vi "Photoeye.vi"(11 "Update":bool) -> (3 "BeamBroken?":bool)   [LabVIEW 2015]
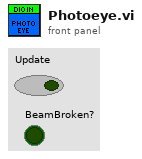
[diagram p1: front panel]
types:
  T1 = typedef "WPI_DigitalInputDevRef.ctl" = cluster{"DevStatus":errorcluster, "DIO Channel":T2}
  T2 = typedef "FPGA_DIOChannel.ctl" = enum8{"DIO 0", "DIO 1", "DIO 2", "DIO 3", "DIO 4", "DIO 5", "DIO 6", "DIO 7", "DIO 8", "DIO 9", "DIO MXP 0", "DIO MXP 1", "DIO MXP 2", "DIO MXP 3", "DIO MXP 4", "DIO MXP 5", "DIO MXP 6", "DIO MXP 7", "DIO MXP 8", "DIO MXP 9", "DIO MXP 10", "DIO MXP 11", "DIO MXP 12", "DIO MXP 13", "DIO MXP 14", "DIO MXP 15", "Invalid"}
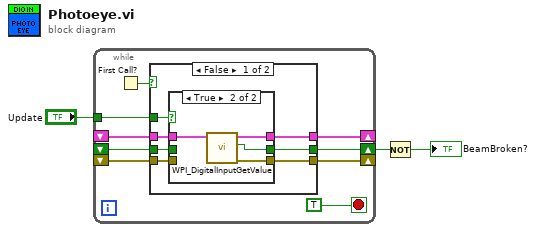
[diagram p0: block diagram]
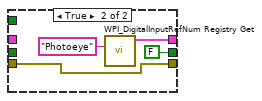
[diagram p3: hidden frame]
diagram:
  n1 = while {
    tunnel: "Update" -> [w10]
    shift-right: [w9] -> _
    shift-left: _ -> [w8]
    shift-right: [w7] -> w2
    shift-left: _ -> [w6]
    shift-right: [w5] -> _
    shift-left: _ -> [w4]
    stop <- TRUE stop-if-true
    n2 = First Call?() -> (First Call?: T/F=w11:bool)
    n3 = case shown="False" w11 {
      tunnel: w10 -> [w19 _]
      tunnel: [w18 w28] -> w9
      tunnel: w8 -> [w17 _]
      tunnel: [w16 FALSE ("Value")] -> w7
      tunnel: w6 -> [w15 _]
      tunnel: [w14 w27] -> w5
      tunnel: w4 -> [w13 w27]
      frame False {
        n4 = case shown="True" w19 {
          tunnel: [w22 w25] -> w18
          tunnel: w17 -> [w22 w26]
          tunnel: [w21 w23] -> w16
          tunnel: w15 -> [w21 _]
          tunnel: [w20 w24] -> w14
          tunnel: w13 -> [w20 _]
          frame False {
          }
          frame True {
            n5 = call <vilib>:"WPI_DigitalInputGetValue.vi"("DigitalInputDevRef"=w26) -> ("error out"=w24:errorcluster, "Value"=w23:bool, "DigitalInputDevRef"=w25:T1)  [unwired: 8 in]
          }
        }
      }
      frame True {
        n6 = call <vilib>:"WPI_DigitalInputRefNum Registry Get.vi"("refnum name"="Photoeye") -> ("DigitalInputDevRef"=w28:T1)  [unwired: 9 in, 1 out]
      }
    }
  }
  n7 = Not(x=w2) -> (.not. x?=→"BeamBroken?":bool)
